vi "Point Data Updated.vi"(8 "error in":errorcluster, 9 "Data":variant, 10 "Point Ident":string, 11 "Series Actor in":refnum<class "Series Actor.lvclass">) -> (0 "error out":errorcluster, 3 "Series Actor out":refnum<class "Series Actor.lvclass">)   [LabVIEW 2023]
uses:
  Series Actor.lvclass
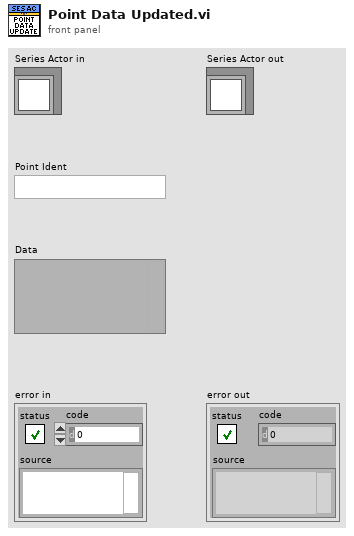
[diagram p1: front panel]
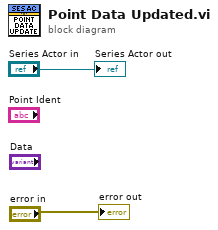
[diagram p0: block diagram]
diagram:
  "error out" <- "error in"
  "Series Actor out" <- "Series Actor in"
